vi "CollectData.vi"(8 "error in (no error)":errorcluster, 11 "Advanced_DMD in":refnum<class "Advanced_DMD.lvclass">) -> (0 "error out":errorcluster, 3 "Advanced_DMD out":refnum<class "Advanced_DMD.lvclass">)   [LabVIEW 2013, in "Advanced_DMD.lvclass"]
uses:
  Advanced_DMD.lvclass
  Device/Device.lvclass
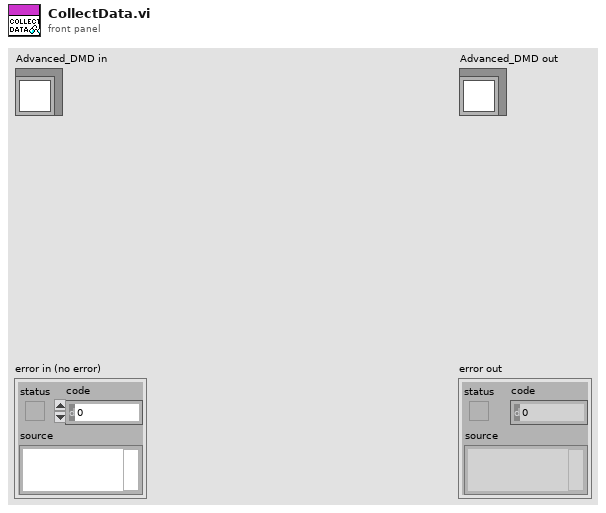
[diagram p1: front panel]
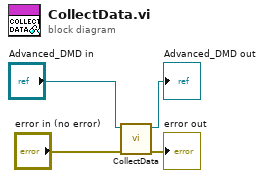
[diagram p0: block diagram]
diagram:
  n1 = call-parent "CollectData.vi"("error in (no error)"="error in (no error)", "Device in"="Advanced_DMD in") -> ("error out"=→"error out":errorcluster, "Device out"=→"Advanced_DMD out":refnum<class "Advanced_DMD.lvclass">)  [unwired: 8 in]
